vi "Data Access Server.vi"() -> ()   [LabVIEW 2019, in "OPC UA Demo.lvlib"]
doc: "Demonstrates the use of the <B>OPC UA Data Access Server</B> VIs to programmatically create an OPC UA server."
uses:
  OPC UA Demo.lvlib
  <vilib>/OPCUA/controls/Supported Security Policies.ctl
  <vilib>/OPCUA/controls/Data Type.ctl
  <vilib>/OPCUA/server/Write Int32.vi
  <vilib>/OPCUA/server/Read Int32.vi
  <vilib>/OPCUA/server/Write Bool.vi
  <vilib>/OPCUA/NI OPC UA Server.lvlib
panel:
  in  "value":bool
  in  "supported security policies (None)":T1={"None"=TRUE, "Sign with Basic128Rsa15"=TRUE, "Sign and Encrypt with Basic128Rsa15"=TRUE, "Sign with Basic256"=TRUE, "Sign and Encrypt with Basic256"=TRUE}
  out "Device.Node.Set Point":i32
  out "Device.Node":i32
  out "server endpoint URL":string
  in  "stop":bool
  # "Overview: Demonstrates the use of the OPC UA Server VIs to programmatically create an OPC UA server.\nRequirements: \n1. LabVIEW OPC UA Toolkit\n2. Run this VI on RT targets or Windows\nInstructions:\n1. Specify supported security policies (None).\n2. Run the VI.\n3. Run Client.vi in OPC UA Demo.lvproj."
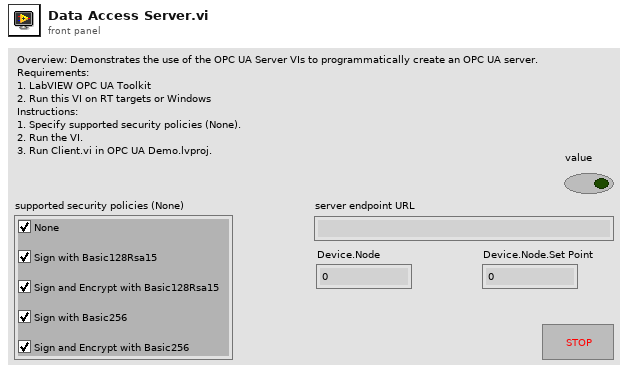
[diagram p1: front panel]
types:
  T1 = typedef "Supported Security Policies.ctl" = cluster{"None":bool, "Sign with Basic128Rsa15":bool, "Sign and Encrypt with Basic128Rsa15":bool, "Sign with Basic256":bool, "Sign and Encrypt with Basic256":bool}
  T2 = typedef "Data Type.ctl" = u16
  T3 = cluster{"name":string, "data type":T2, "access level":u16, "description":string}
  T4 = typedef "OPC UA Server Refnum.ctl" = refnum<k21>
  T5 = typedef "NodeId.ctl" = string
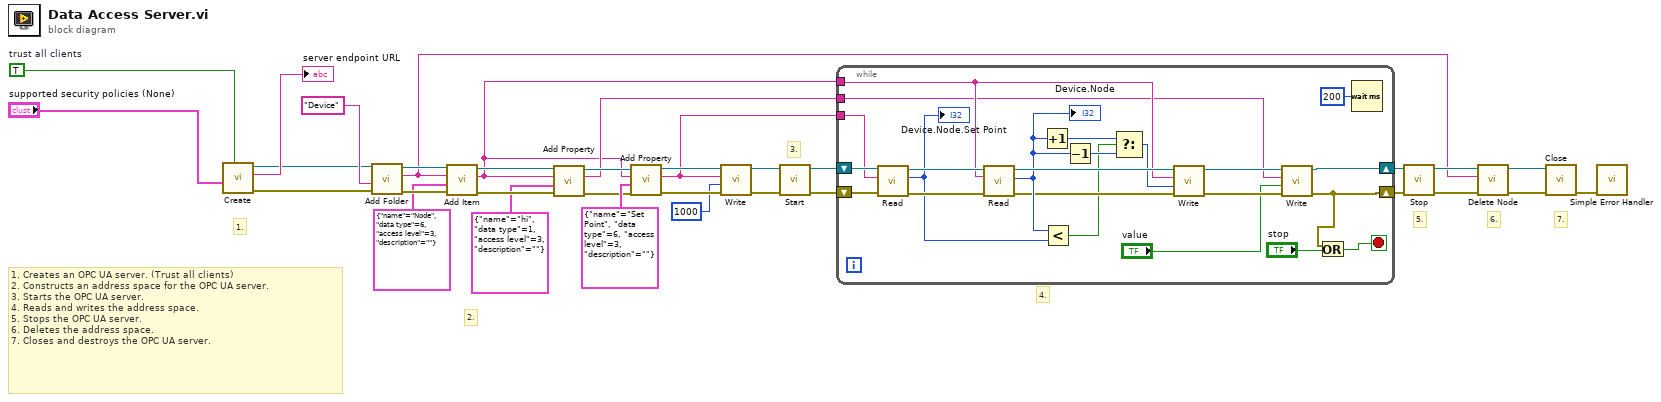
[diagram p0: block diagram]
diagram:
  w8 = TRUE  # trust all clients
  # "1. Creates an OPC UA server. (Trust all clients)\n2. Constructs an address space for the OPC UA server.\n3. Starts the OPC UA server.\n4. Reads and writes the address space.\n5. Stops the OPC UA server.\n6. Deletes the address space.\n7. Closes and destroys the OPC UA server."
  # "7."
  # "6."
  # "5."
  # "4."
  # "3."
  # "2."
  # "1."
  n1 = call <vilib>:"Create.vi"("trust all clients (F)"=w8, "supported security policies (None)"="supported security policies (None)") -> ("error out"=w9:errorcluster, "server endpoint URL"=→"server endpoint URL":string, "OPC UA server refnum out"=w10:T4)  [unwired: 7 in]
  n2 = call <vilib>:"Add Folder.vi"("error in (no error)"=w9, "folder name"="Device", "OPC UA server refnum in"=w10) -> ("error out"=w32:errorcluster, "folder node ID"=w22:T5, "OPC UA server refnum out"=w33:T4)  [unwired: 5 in]
  n3 = call <vilib>:"Add Item.vi"("error in (no error)"=w32, "item"=T3 {"name"="Node", "data type"=6, "access level"=3, "description"=""}, "parent folder node ID"=w22, "OPC UA server refnum in"=w33) -> ("error out"=w7:errorcluster, "item node ID"=w1:T5, "OPC UA server refnum out"=w6:T4)  [unwired: 3 in, 1 out]
  n4 = call <vilib>:"Add Property.vi"("error in (no error)"=w7, "property"=T3 {"name"="hi", "data type"=1, "access level"=3, "description"=""} ("item"), "item node ID"=w1, "OPC UA server refnum in"=w6) -> ("error out"=w4:errorcluster, "property node ID"=w3:T5, "OPC UA server refnum out"=w5:T4)  [unwired: 3 in, 1 out]
  n5 = call <vilib>:"Add Property.vi"("error in (no error)"=w4, "property"=T3 {"name"="Set Point", "data type"=6, "access level"=3, "description"=""}, "item node ID"=w1, "OPC UA server refnum in"=w5) -> ("error out"=w23:errorcluster, "property node ID"=w15:T5, "OPC UA server refnum out"=w24:T4)  [unwired: 3 in, 1 out]
  n6 = call-poly <vilib>:"Write.vi"("error in (no error)"=w23, "value"=1000, "node ID"=w15, "OPC UA server refnum in"=w24) -> ("error out"=w14:errorcluster, "OPC UA server refnum out"=w13:T4)  [unwired: 5 in, 1 out]
  n7 = call <vilib>:"Start.vi"("error in (no error)"=w14, "OPC UA server refnum in"=w13) -> ("error out"=w11:errorcluster, "OPC UA server refnum out"=w12:T4)  [unwired: 7 in, 1 out]
  n8 = while {
    tunnel: w1 -> [w49]
    shift-right: [w39] -> w28
    shift-left: w12 -> [w53]
    shift-right: [w37] -> w26
    shift-left: w11 -> [w55]
    tunnel: w15 -> [w52]
    tunnel: w3 -> [w36]
    stop <- w42 stop-if-true
    n9 = call-poly <vilib>:"Read.vi"("error in (no error)"=w55, "node ID"=w52, "OPC UA server refnum in"=w53) -> ("error out"=w50:errorcluster, "value"=w48:i32, "OPC UA server refnum out"=w56:T4)  [unwired: 4 in, 2 out]
    "Device.Node.Set Point" <- w48
    n10 = call-poly <vilib>:"Read.vi"("error in (no error)"=w50, "node ID"=w49, "OPC UA server refnum in"=w56) -> ("error out"=w43:errorcluster, "value"=w45:i32, "OPC UA server refnum out"=w51:T4)  [unwired: 4 in, 2 out]
    "Device.Node" <- w45
    n11 = Increment(x=w45) -> (x+1=w47:i32)
    n12 = Less?(x=w45, y=w48) -> (x < y?=w35:bool)
    n13 = Decrement(x=w45) -> (x-1=w46:i32)
    n14 = Select(t=w47, s=w35, f=w46) -> (s? t:f=w44:i32)
    n15 = call-poly <vilib>:"Write.vi"("error in (no error)"=w43, "value"=w44, "node ID"=w49, "OPC UA server refnum in"=w51) -> ("error out"=w38:errorcluster, "OPC UA server refnum out"=w40:T4)  [unwired: 5 in, 1 out]
    n16 = call-poly <vilib>:"Write.vi"("error in (no error)"=w38, "value"="value", "node ID"=w36, "OPC UA server refnum in"=w40) -> ("error out"=w37:errorcluster, "OPC UA server refnum out"=w39:T4)  [unwired: 5 in, 1 out]
    n17 = Or(x=w37, y="stop") -> (x .or. y?=w42:bool)
    n18 = Wait (ms)(milliseconds to wait=u32 200) -> ()  [unwired: 1 out]
  }
  n19 = call <vilib>:"Stop.vi"("error in (no error)"=w26, "OPC UA server refnum in"=w28) -> ("error out"=w25:errorcluster, "OPC UA server refnum out"=w27:T4)  [unwired: 8 in]
  n20 = call <vilib>:"Delete Node.vi"("error in (no error)"=w25, "node ID"=w22, "OPC UA server refnum in"=w27) -> ("error out"=w29:errorcluster, "OPC UA server refnum out"=w30:T4)  [unwired: 7 in]
  n21 = call <vilib>:"Close.vi"("error in (no error)"=w29, "OPC UA server refnum in"=w30) -> ("error out"=w18:errorcluster)  [unwired: 9 in]
  n22 = call <vilib>:"Simple Error Handler.vi"("error in (no error)"=w18) -> ()  [unwired: 4 in, 5 out]
